vi "Exponential_Rolling_Average.vi"(9 "Previous Value":dbl, 10 "Weight":dbl, 11 "Input Value":dbl) -> (2 "Weighted Value":dbl)   [LabVIEW 2012]
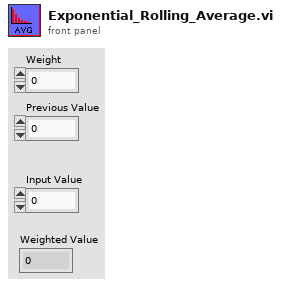
[diagram p1: front panel]
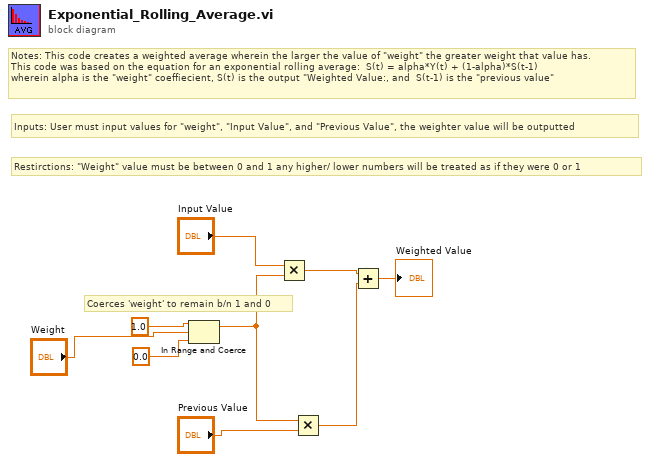
[diagram p0: block diagram]
diagram:
  # "Inputs: User must input values for \"weight\", \"Input Value\", and \"Previous Value\", the weighter value will be outputted"
  # "Restirctions: \"Weight\" value must be between 0 and 1 any higher/ lower numbers will be treated as if they were 0 or 1"
  # "Coerces 'weight' to remain b/n 1 and 0"
  # "Notes: This code creates a weighted average wherein the larger the value of \"weight\" the greater weight that value has.\nThis code was based on the equation for an exponential rolling average:  S(t) = alpha*Y(t) + (1-alpha)*S(t-1)\nwherein alpha is the \"weight\" coeffiecient, S(t) is the output \"Weighted Value:, and  S(t-1) is the \"previous value\""
  n1 = In Range and Coerce(upper limit=1.0, x="Weight", lower limit=0.0) -> (coerced(x)=w4:dbl)  [unwired: 1 out]
  n2 = Multiply(x="Input Value", y=w4) -> (x*y=w2:dbl)
  n3 = Multiply(x=w4, y="Previous Value") -> (x*y=w3:dbl)
  n4 = Add(x=w2, y=w3) -> (x+y=→"Weighted Value":dbl)
